vi "Shut Down Server.vi"(10 "name or relative path":string="TestScripts", 11 "Sequence path":path=path "C:/Func Jobs/SnapOn/ModisEdge/Scanner/Test Sequence/ModisEdgeScanner.seq") -> ()   [LabVIEW 2015]
panel:
  out "error out":errorcluster
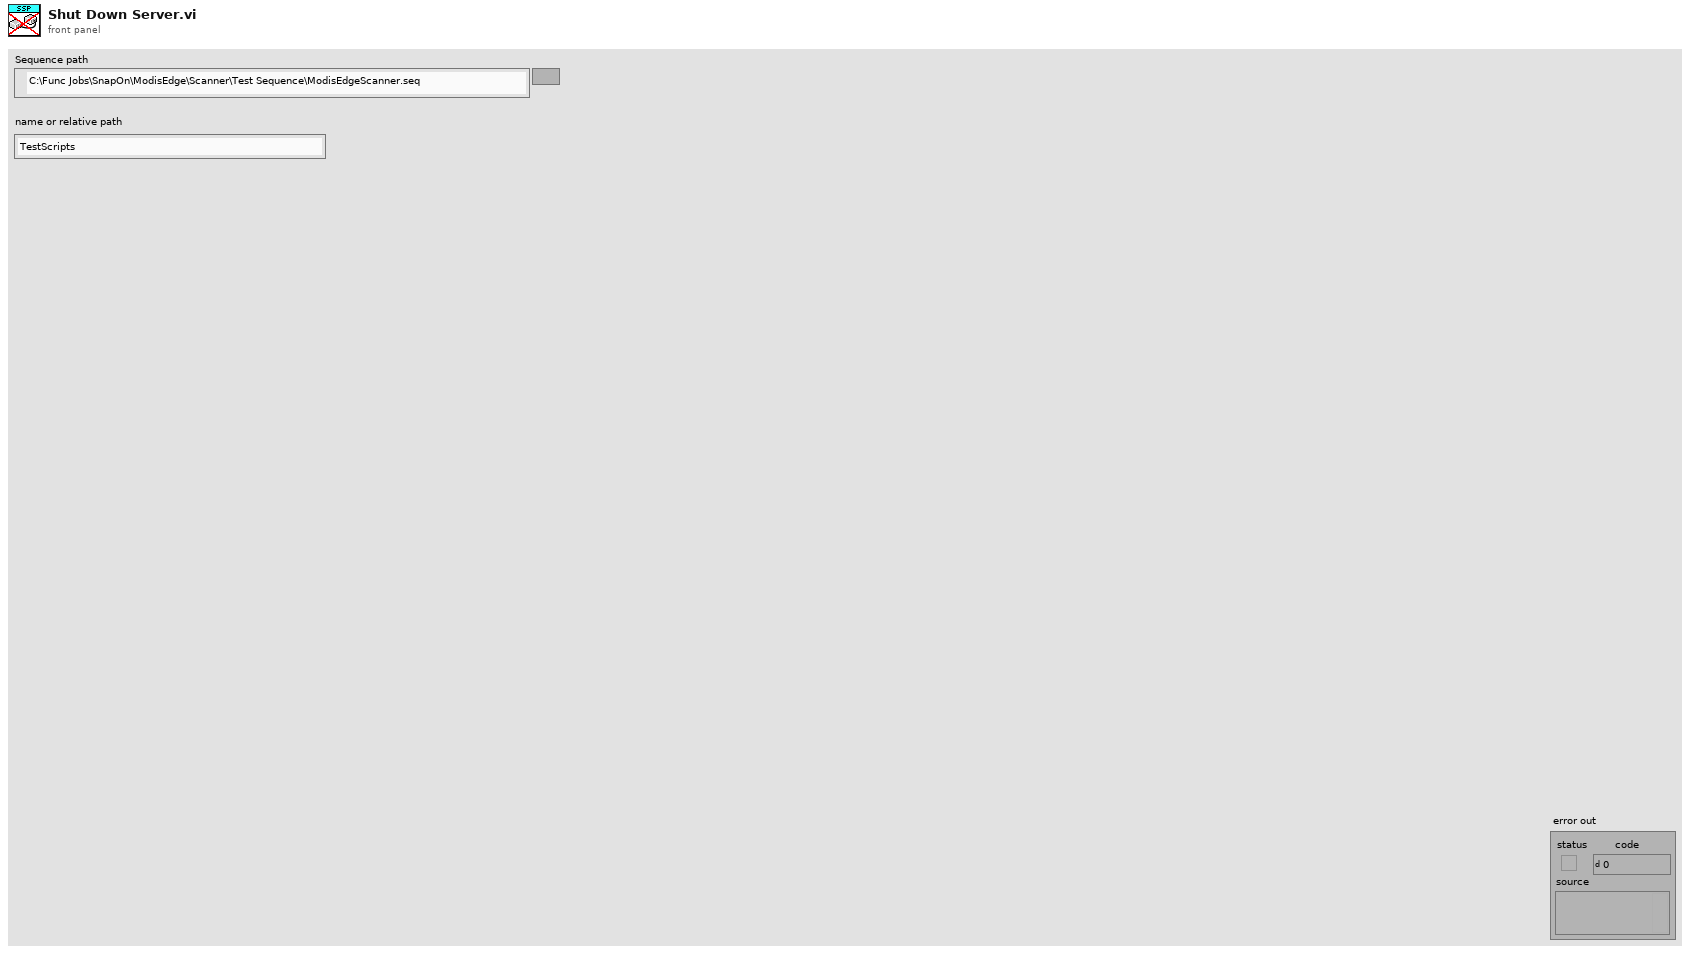
[diagram p1: front panel]
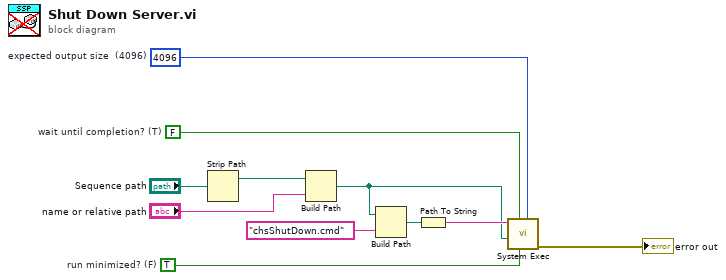
[diagram p0: block diagram]
diagram:
  w1 = TRUE  # run minimized? (F)
  w11 = FALSE  # wait until completion? (T)
  w2 = u32 4096  # expected output size  (4096)
  n1 = Strip Path(path="Sequence path") -> (stripped path=w5:path)  [unwired: 1 out]
  n2 = Build Path(base path=w5, name or relative path="name or relative path") -> (appended path=w3:path)
  n3 = Build Path(base path=w3, name or relative path="chsShutDown.cmd" ("Command")) -> (appended path=w8:path)
  n4 = Path To String(path=w8) -> (string=w7:string)
  n5 = call <vilib>:"System Exec.vi"("expected output size  (4096)"=w2, "run minimized? (F)"=w1, "wait until completion? (T)"=w11, "working directory"=w3, "command line"=w7) -> ("error out"=→"error out":errorcluster)  [unwired: 3 in, 3 out]
